vi "Execute Value Update Policy.vi"(8 "error in (no error)":errorcluster, 9 "Publish Time":timestamp, 10 "New Topic Value":variant, 11 "BasicSubscription In":refnum<class "BasicSubscription.lvclass">) -> (0 "error out":errorcluster, 3 "BasicSubscription Out":refnum<class "BasicSubscription.lvclass">)   [LabVIEW 2018, in "MVA Framework.lvlib" / "SubscriptionPolicy.lvlib" / "BasicSubscription.lvclass"]
doc: "执行值更新策略"
uses:
  BasicSubscription.lvclass
  IMediator/ISubscriptionPolicy/ISubscriptionPolicy.lvclass
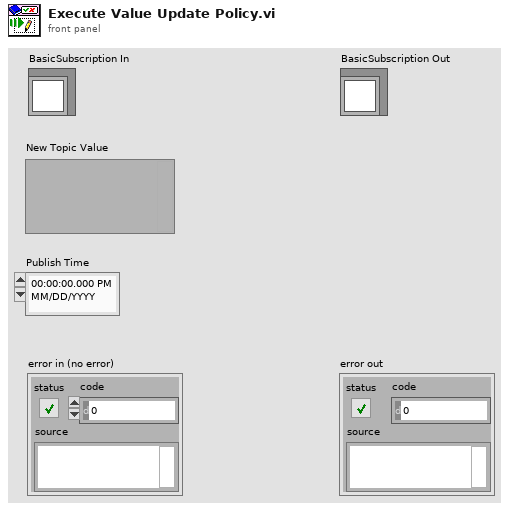
[diagram p1: front panel]
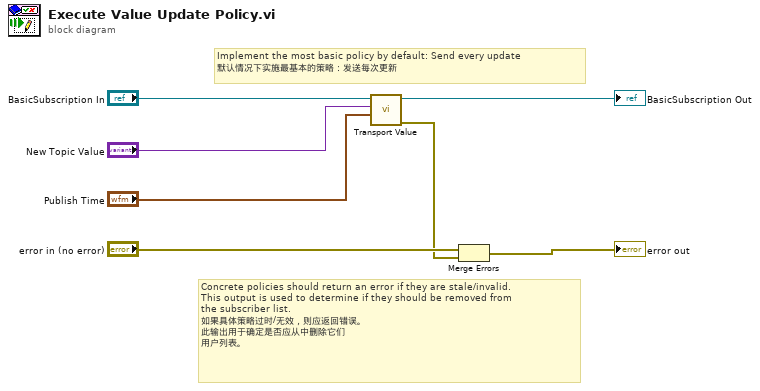
[diagram p0: block diagram]
diagram:
  # "Implement the most basic policy by default: Send every update\n默认情况下实施最基本的策略：发送每次更新"
  # "Concrete policies should return an error if they are stale/invalid.\nThis output is used to determine if they should be removed from\nthe subscriber list.\n如果具体策略过时/无效，则应返回错误。\n此输出用于确定是否应从中删除它们\n用户列表。"
  n1 = call "Transport Value.vi"("Publish Time"="Publish Time", "Value"="New Topic Value", "ISubscriptionPolicy in"="BasicSubscription In") -> ("error out"=w1:errorcluster, "ISubscriptionPolicy out"=→"BasicSubscription Out":refnum<class "BasicSubscription.lvclass">)  [unwired: 7 in]
  n2 = Merge Errors("error in (no error)", w1) -> (→"error out":errorcluster)
